vi "flat disorder.vi"(8 "error in":errorcluster, 10 "level":dbl=1.0, 11 "Points":i32=10) -> (0 "error out":errorcluster, 3 "disorder":dbl[](array[numeric]))   [LabVIEW 2023]
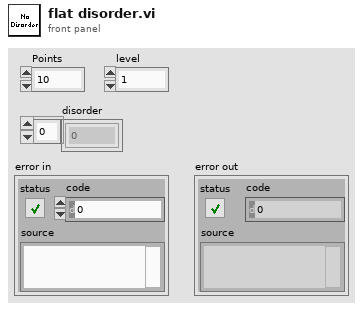
[diagram p1: front panel]
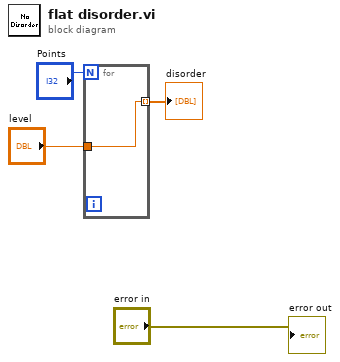
[diagram p0: block diagram]
diagram:
  n1 = for {
    N: "Points" -> [_]
    tunnel: [w5] -> w3 mode=indexing
    tunnel: "level" -> [w5]
  }
  "disorder" <- w3
  "error out" <- "error in"
